vi "Status.vi"(8 "error in (no error)":errorcluster, 11 "SS P100 Settings In":T1) -> (0 "error out":errorcluster, 1 "Connection Error":bool, 2 "Running":bool, 3 "SS P100 Settings Out":T1, 4 "Power":dbl, 5 "Amplitude":dbl)   [LabVIEW 2018, in "Sonic Systems P100.lvlib"]
uses:
  Sonic Systems P100.lvlib
  Sonic Systems P100 Settings.ctl
  <vilib>/regexp/Match Regular Expression.xnode
  support/Support Library.lvlib
panel:
  out "read buffer":string
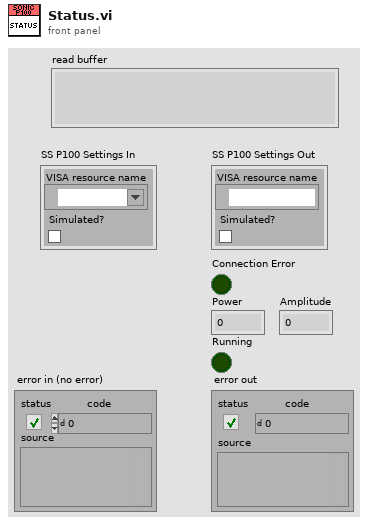
[diagram p1: front panel]
types:
  T1 = typedef "Sonic Systems P100.lvlib/Sonic Systems P100 Settings.ctl" = cluster{"VISA resource name":refnum<visa-resource-name>, "Simulated?":bool}
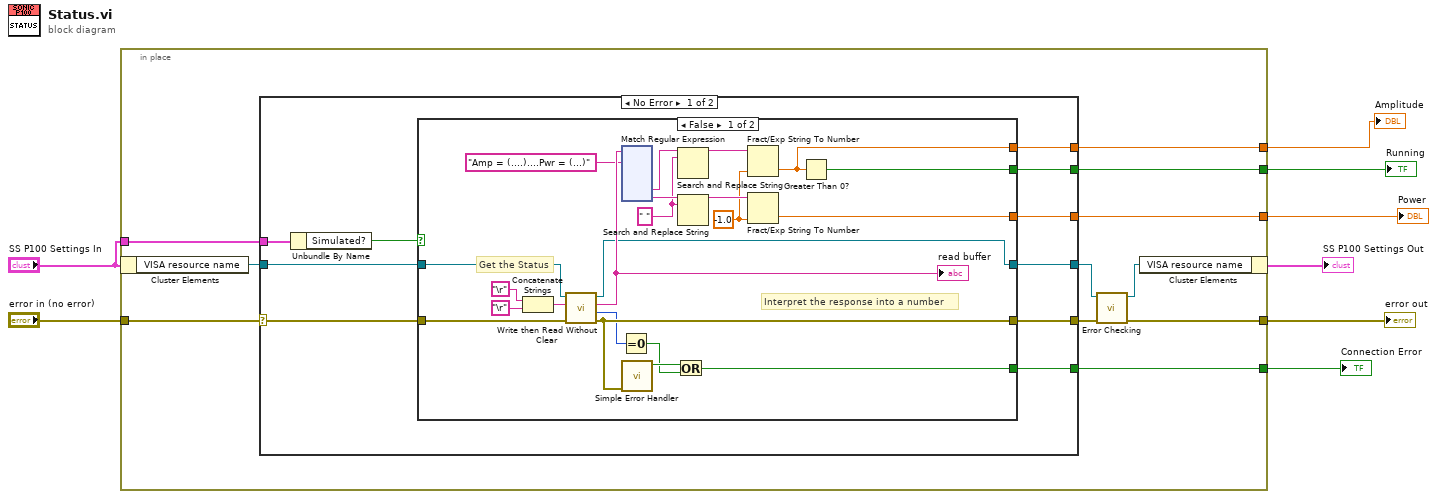
[diagram p0: block diagram]
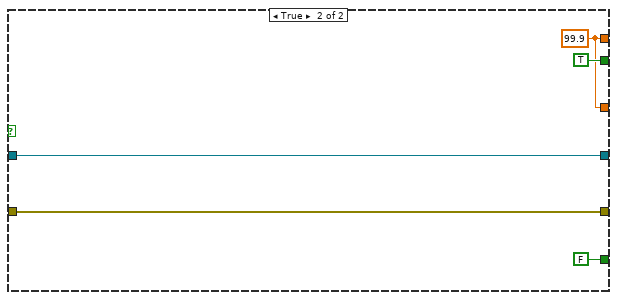
[diagram p2: hidden frame]
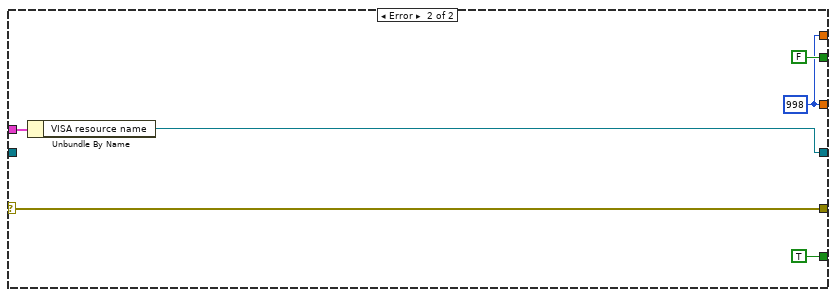
[diagram p3: hidden frame]
diagram:
  n1 = in-place {
    in-place-border: "error in (no error)" -> [w19]
    in-place-border: [w16] -> w7
    in-place-border: "SS P100 Settings In" -> [w15]
    in-place-border: [w12] -> w4
    in-place-border: [w10] -> w2
    in-place-border: [w11] -> w3
    in-place-border: [w9] -> w1
    n2 = in-place-cluster #1("SS P100 Settings In") -> ("VISA resource name"=w14:refnum<visa-resource-name>)
    n3 = case shown="No Error" w19 {
      selector: w19 -> [w29 w179]
      tunnel: w15 -> [w27 w178]
      tunnel: [w28 w179] -> w17
      tunnel: [w26 w177] -> w18
      tunnel: [w24 TRUE] -> w12
      tunnel: [w23 FALSE] -> w11
      tunnel: w14 -> [w22 _]
      tunnel: [w21 w174] -> w10
      tunnel: [w20 w174] -> w9
      frame No Error {
        n4 = Unbundle By Name(w27) -> ("Simulated?"=w25:bool)
        n5 = case shown="False" w25 {
          tunnel: w29 -> [w48 w173]
          tunnel: [w46 w173] -> w28
          tunnel: [w50 w172] -> w26
          tunnel: w22 -> [w49 w172]
          tunnel: [w44 FALSE] -> w24
          tunnel: [w38 TRUE] -> w23
          tunnel: [w36 w169] -> w21
          tunnel: [w37 w169] -> w20
          frame False {
            w30 = -1.0 ("default (0 DBL)")
            w33 = " " ("search string")
            # "Interpret the response into a number"
            # "Get the Status"
            n6 = Concatenate Strings("\r", "\r") -> (w39:string)
            n7 = call "Write then Read Without Clear.vi"("error in"=w48, "write buffer"=w39, "VISA resource name in"=w49) -> ("error out"=w46:errorcluster, "Bytes at Port"=w43:u32, "read buffer"=w51:string, "VISA resource name out"=w50:refnum<visa-resource-name>)  [unwired: 5 in]
            "read buffer" <- w51
            n8 = Equal To 0?(x=w43) -> (x = 0?=w42:bool)
            n9 = xnode "Match Regular Expression"("input string"=w51, "regular expression"="Amp = (....)....Pwr = (...)") -> ("submatch 1"=w34:string, "submatch 2"=w35:string)  [unwired: 4 in, 5 out]
            n10 = call <vilib>:"Simple Error Handler.vi"("error in (no error)"=w46) -> ("error?"=w45:bool)  [unwired: 4 in, 4 out]
            n11 = Or(x=w45, y=w42) -> (x .or. y?=w44:bool)
            n12 = Search and Replace String(input string=w34, search string=w33) -> (result string=w32:string)  [unwired: 6 in, 3 out]
            n13 = Search and Replace String(input string=w35, search string=w33) -> (result string=w31:string)  [unwired: 6 in, 3 out]
            n14 = Fract/Exp String To Number(string=w32, default (0 dbl)=w30) -> (number=w36:dbl)  [unwired: 2 in, 1 out]
            n15 = Fract/Exp String To Number(string=w31, default (0 dbl)=w30) -> (number=w37:dbl)  [unwired: 2 in, 1 out]
            n16 = Greater Than 0?(x=w36) -> (x > 0?=w38:bool)
          }
          frame True {
            w169 = 99.9
          }
        }
      }
      frame Error {
        w174 = 998
        n17 = Unbundle By Name(w178) -> ("VISA resource name"=w177:refnum<visa-resource-name>)
      }
    }
    n18 = call "Error Checking.vi"("error in (no error)"=w17, "VISA resource name"=w18) -> ("error out"=w16:errorcluster, "VISA resource name"=w13:refnum<visa-resource-name>)  [unwired: 7 in, 1 out]
    n19 = in-place-cluster #1("VISA resource name"=w13) -> (→"SS P100 Settings Out":T1)
  }
  "error out" <- w7
  "Connection Error" <- w4
  "Power" <- w1
  "Running" <- w3
  "Amplitude" <- w2
